vi "Count_if_Subtrack_Is_Enough_for_Cost_F()-4.vi"(3 "[IN] Minimal Subtrack Length \n(Points without problems) for\nMaking Desicion":i32, 4 "[IN] Index of Problem \nPoint Inside Track":i32, 5 "[IN] Dot Statuses in Track":i16[](array[numeric])) -> (0 "[OUT] Index of Last \nPoint in Track":i32, 2 "[OUT] It's enough to make\nconclusion using subtrack":bool)   [LabVIEW 2017]
doc: "Subprogram calculates how many points before problem point under revision and after (before further problem points) are in the track\n\"101\" points are treated as points without problems..."
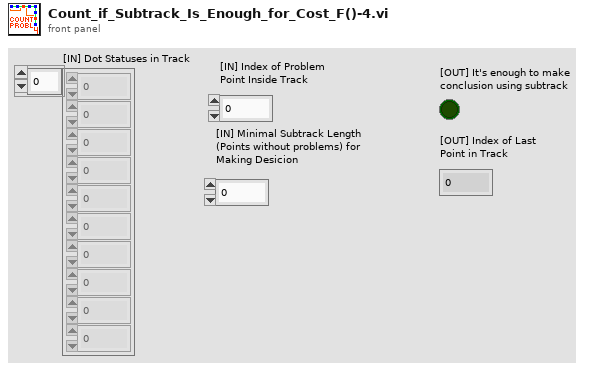
[diagram p1: front panel]
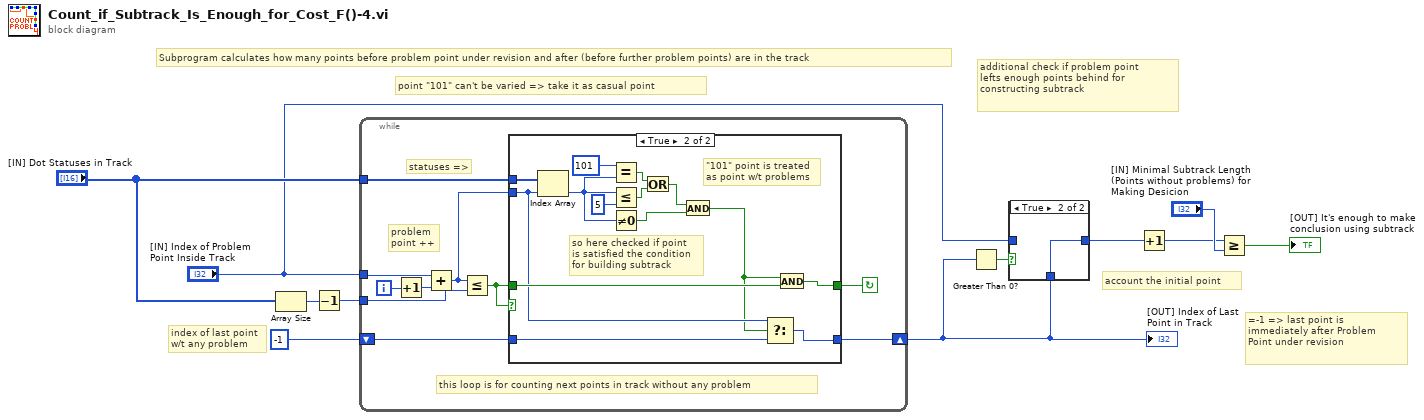
[diagram p0: block diagram]
diagram:
  # "point \"101\" can't be varied => take it as casual point"
  # "account the initial point"
  # "additional check if problem point \nlefts enough points behind for \nconstructing subtrack"
  # "=-1 => last point is\nimmediately after Problem \nPoint under revision"
  # "Subprogram calculates how many points before problem point under revision and after (before further problem points) are in the track"
  # "index of last point\nw/t any problem"
  n1 = Array Size(array="[IN] Dot Statuses in Track") -> (size(s)=w11:i32)
  n2 = Decrement(x=w11) -> (x-1=w10:i32)
  n3 = while {
    tunnel: w10 -> [w19]
    tunnel: "[IN] Index of Problem \nPoint Inside Track" -> [w12]
    tunnel: "[IN] Dot Statuses in Track" -> [w18]
    shift-right: [w13] -> w3
    shift-left: -1 -> [w14]
    i -> [w21]
    stop <- w15 continue-if-true
    # "statuses =>"
    # "problem \npoint ++"
    # "this loop is for counting next points in track without any problem"
    n4 = Increment(x=w21) -> (x+1=w20:i32)
    n5 = Add(x=w12, y=w20) -> (x+y=w17:i32)
    n6 = Less Or Equal?(x=w17, y=w19) -> (x <= y?=w16:bool)
    n7 = case shown="True" w16 {
      tunnel: w18 -> [_ w37]
      tunnel: w17 -> [_ w30]
      tunnel: w16 -> [w23 w33]
      tunnel: [w23 w34] -> w15
      tunnel: w14 -> [w22 w31]
      tunnel: [w22 w32] -> w13
      frame False {
        # "it's last point in subtrack"
      }
      frame True {
        # "so here checked if point \nis satisfied the condition \nfor building subtrack"
        # "\"101\" point is treated \nas point w/t problems"
        n8 = Index Array(array=w37, index=w30) -> (element=w28:i16)
        n9 = Equal?(x=i16 101, y=w28) -> (x = y?=w26:bool)
        n10 = Less Or Equal?(x=w28, y=i16 5) -> (x <= y?=w25:bool)
        n11 = Not Equal To 0?(x=w28) -> (x != 0?=w35:bool)
        n12 = Or(x=w26, y=w25) -> (x .or. y?=w24:bool)
        n13 = And(x=w24, y=w35) -> (x .and. y?=w29:bool)
        n14 = Select(t=w30, s=w29, f=w31) -> (s? t:f=w32:i32)
        n15 = And(x=w29, y=w33) -> (x .and. y?=w34:bool)
      }
    }
  }
  "[OUT] Index of Last \nPoint in Track" <- w3
  n16 = Greater Than 0?(x=w3) -> (x > 0?=w5:bool)
  n17 = case shown="True" w5 {
    tunnel: "[IN] Index of Problem \nPoint Inside Track" -> [w38 _]
    tunnel: [w38 w39] -> w4
    tunnel: w3 -> [_ w39]
    frame False {
    }
    frame True {
    }
  }
  n18 = Increment(x=w4) -> (x+1=w6:i32)
  n19 = Greater Or Equal?(x=w6, y="[IN] Minimal Subtrack Length \n(Points without problems) for\nMaking Desicion") -> (x >= y?=→"[OUT] It's enough to make\nconclusion using subtrack":bool)
